vi "produce_data.vi"(6 "Queues":T1, 7 "Producer LD Data In":T3[](array[typedef]), 8 "error in (no error)":errorcluster, 9 "NumReadAddresses":i32, 10 "ScansPerRead Out":i32, 11 "Ref":i32) -> (0 "error out":errorcluster, 3 "Handle Out":i32, 5 "Loop Data Out":T3[](array[typedef]))   [LabVIEW 2025, in "LabJackEKG.lvlib"]
uses:
  LabJackEKG.lvlib
  Tests/StreamProducerLoopData.ctl
  Typedefs/LabJackGlobalResources.ctl
  Typedefs/CounterQueues.ctl
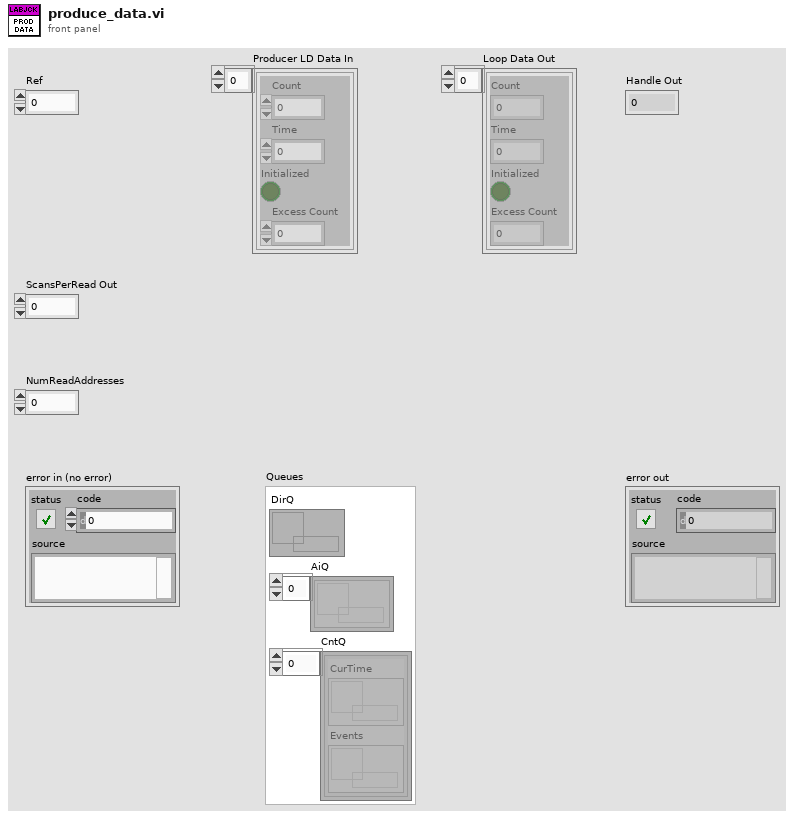
[diagram p1: front panel]
types:
  T1 = typedef "LabJackEKG.lvlib/LabJackGlobalResources.ctl" = cluster{"DirQ":refnum<queue>, "AiQ":refnum<queue>[], "CntQ":T2[]}
  T2 = typedef "LabJackEKG.lvlib/CounterQueues.ctl" = cluster{"CurTime":refnum<queue>, "Events":refnum<queue>}
  T3 = typedef "LabJackEKG.lvlib/StreamProducerLoopData.ctl" = cluster{"Count":i64, "Time":dbl, "Initialized":bool, "Excess Count":i64}
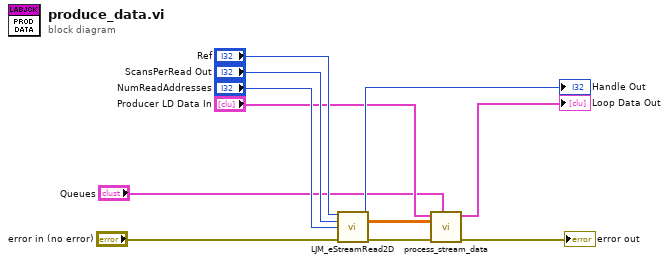
[diagram p0: block diagram]
diagram:
  n1 = call <vilib>:"LJM_eStreamRead2D.vi"("Handle In"="Ref", "ScansPerRead"="ScansPerRead Out", "NumAddresses"="NumReadAddresses", "error in"="error in (no error)") -> ("Handle Out"=→"Handle Out":i32, "aData Out"=w2:dbl[][], "error out"=w7:errorcluster)  [unwired: 7 in, 2 out]
  n2 = call "process_stream_data.vi"("Queues"="Queues", "error in (no error)"=w7, "aData Out"=w2, "Loop Data In"="Producer LD Data In") -> ("error out"=→"error out":errorcluster, "Loop Data Out"=→"Loop Data Out":T3[])  [unwired: 6 in]
